vi "Write Power FIFO Direct Dispatch.vi"(4 "T_Out":u64, 6 "T0":u64, 8 "error in (no error)":errorcluster, 9 "Timeout (ms)":i32=100, 10 "Data In":T1[](array[typedef])=[{"measurement"=[], "dT"=0.0, "Timestamp"=0}, {"measurement"=[], "dT"=0.0, "Timestamp"=0}], 11 "CIFTag in":refnum<class "CIFChannels.lvclass">) -> (0 "error out":errorcluster, 1 "timed out?":bool, 2 "Data Out":T1[](array[typedef]), 3 "CIFTag out":refnum<class "CIF_NIChn_Fifo_Power.lvclass">)   [LabVIEW 2021, in "CIF_NIChn_Fifo_Power.lvclass"]
uses:
  CIF_NIChn_Fifo_Power.lvclass
  D:/dev/CIF-LVCore/src/Channels/CIFChannels/CIFChannels.lvclass
  D:/dev/CIF-LVCore/src/Channels/CIF_NIChn/NIChn/CIF_NIChn.lvclass
  CIFChannels/CIFChannels.lvclass
  ChannelCommon/typedef/Datatype Waveform.ctl
  CIFChannels/CIFChannels.lvclass/CIFChannels.ctl
  CIF_NIChn_Fifo_Power.lvclass/CIF_NIChn_Fifo_Power.ctl
  ChannelCommon/CIFFIFO/CIFfifo.lvclass/CIFfifo.ctl
  NIChn/CIF_NIChn.lvclass/CIF_NIChn.ctl
  ChannelCommon/CIFFIFO/Accessors/Read Length.vi
  <vilib>/CIFChannels/SubVIs/Get dll Path.vi
  ChannelCommon/CIFFIFO/Utilities/Update Header.vi
  ChannelCommon/Utilities/Flatten Header.vi
  ChannelCommon/Flatten/Waveform Flatten.vi
  ChannelCommon/CIFFIFO/Accessors/Write T0.vi
  ChannelCommon/CIFFIFO/Accessors/Write T_Out.vi
  ChannelCommon/CIFFIFO/Accessors/Write Payload Length.vi
  ChannelCommon/CIFFIFO/Accessors/Read Header.vi
  ChannelCommon/CIFFIFO/Accessors/Write Header.vi
  CIFChannels/Accessors/Read ClockID.vi
  ChannelCommon/Flatten/Waveform Flatten.vi/e2488641-f297-4923-bbd0-3c2628a14485.vi
  ChannelCommon/Flatten/Waveform Flatten.vi/b4043d5f-ec85-461b-bf30-5d9c9f378a85.vi
  ChannelCommon/Flatten/Waveform Flatten.vi/7a03eb27-3fd6-4af7-b359-0d2263a4e3bc.vi
  CIFCore/Common/Utilities/Append Error Location.vi
  ChannelCommon/Flatten/Waveform Flatten.vi/e2488641-f297-4923-bbd0-3c2628a14485.vi/c28b0ead-42ad-4072-80a2-aca7f2bd7ce3.vi
  ChannelCommon/Flatten/Waveform Flatten.vi/b4043d5f-ec85-461b-bf30-5d9c9f378a85.vi/c28b0ead-42ad-4072-80a2-aca7f2bd7ce3.vi
  ChannelCommon/Flatten/Waveform Flatten.vi/7a03eb27-3fd6-4af7-b359-0d2263a4e3bc.vi/c28b0ead-42ad-4072-80a2-aca7f2bd7ce3.vi
  ChannelCommon/Utilities/Update Time.vi
  NIChn/CIF_NIChn.lvclass
  <vilib>/CIFChannels/CIFChannelCore.lvlib
  ChannelCommon/CIFFIFO/CIFfifo.lvclass
  ChannelCommon/ChannelCommon.lvlib
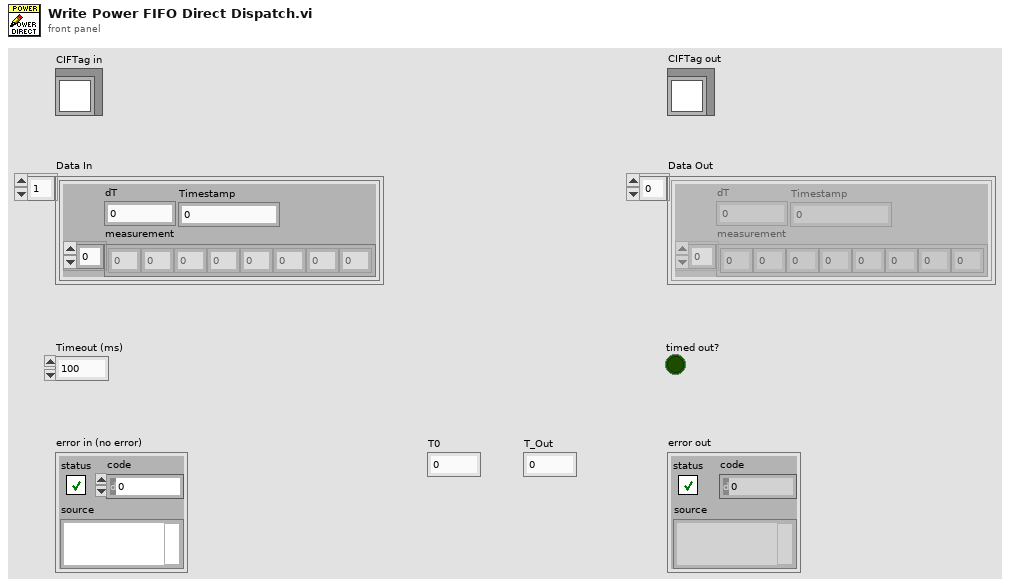
[diagram p1: front panel]
types:
  T1 = typedef "ChannelCommon.lvlib/Datatype Waveform.ctl" = cluster{"measurement":dbl[], "dT":dbl, "Timestamp":u64}
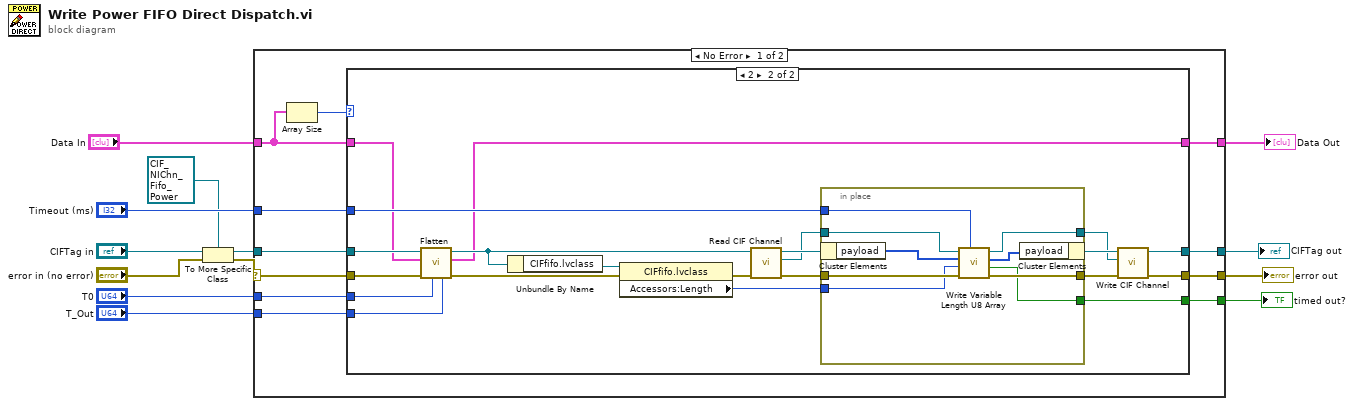
[diagram p0: block diagram]
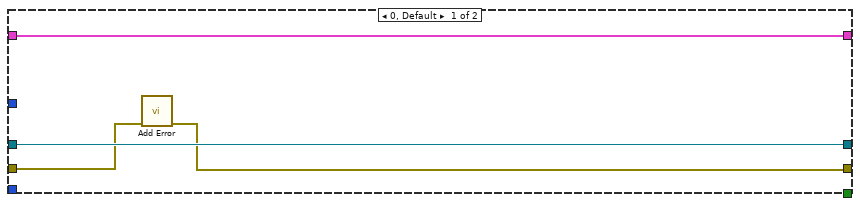
[diagram p2: hidden frame]
diagram:
  n1 = To More Specific Class(target class=refnum<class "CIF_NIChn_Fifo_Power.lvclass"> refnum ("CIFTag in"), reference="CIFTag in", error in="error in (no error)") -> (specific class reference=w5:refnum<class "CIF_NIChn_Fifo_Power.lvclass">, error out=w3:errorcluster)
  n2 = case shown="No Error" w3 {
    selector: w3 -> [w19 w61]
    tunnel: [w21 w61] -> w13
    tunnel: [w23 w60] -> w12
    tunnel: w5 -> [w20 w60]
    tunnel: [w24 _] -> w11
    tunnel: "Timeout (ms)" -> [w22 _]
    tunnel: "T_Out" -> [w17 _]
    tunnel: "T0" -> [w18 _]
    tunnel: "Data In" -> [w14 w59]
    tunnel: [w16 w59] -> w1
    frame No Error {
      n3 = Array Size(array=w14) -> (size(s)=w15:i32)
      n4 = case shown="2" w15 {
        tunnel: [_ w49] -> w24
        tunnel: [w27 w45] -> w23
        tunnel: w22 -> [_ w41]
        tunnel: [w25 w40] -> w21
        tunnel: w20 -> [w27 w37]
        tunnel: w19 -> [w26 w34]
        tunnel: w18 -> [_ w33]
        tunnel: w17 -> [_ w32]
        tunnel: w14 -> [w28 w30]
        tunnel: [w28 w29] -> w16
        frame 0, Default {
          n5 = call "Add Error.vi"("error in (no error)"=w26) -> ("error out"=w25:errorcluster)  [unwired: 10 in]
        }
        frame 2 {
          n6 = call "Flatten.vi"("T_Out"=w32, "T0"=w33, "error in (no error)"=w34, "Data"=w30, "CIFTag in"=w37) -> ("error out"=w35:errorcluster, "Data out"=w29:T1[], "CIFTag out"=w36:refnum<class "CIF_NIChn_Fifo_Power.lvclass">)  [unwired: 4 in]
          n7 = Unbundle By Name(w36) -> ("CIFfifo.lvclass"=w39:refnum<class "CIFfifo.lvclass">)
          n8 = property class="CIFfifo.lvclass"(reference=w39, error in=w35) -> (error out=w38:errorcluster, "Accessors:Length"=w31:u64)  [unwired: 1 out]
          n9 = call "Read CIF Channel.vi"("error in (no error)"=w38, "CIFTag in"=w36) -> ("error out"=w47:errorcluster, "CIF Channel"=w43:refnum<k21>, "CIFTag out"=w48:refnum<class "CIF_NIChn_Fifo_Power.lvclass">)  [unwired: 7 in]
          n10 = in-place {
            in-place-border: w47 -> [w58]
            in-place-border: [w57] -> w44
            in-place-border: [w56] -> w49
            in-place-border: w43 -> [w55]
            in-place-border: [w54] -> w42
            in-place-border: w41 -> [w53]
            in-place-border: w31 -> [w51]
            n11 = in-place-cluster #1(w48) -> ("payload"=w52:u8[])
            n12 = call <vilib>:"Write Variable Length U8 Array.vi"("Timeout (ms)"=w53, "error in"=w58, "numElements"=w51, "U8 Array in"=w52, "CIF Channel in"=w55) -> ("error out"=w57:errorcluster, "Timed out?"=w56:bool, "U8 Array out"=w50:u8[], "CIF Channel out"=w54:refnum<k21>)  [unwired: 3 in]
            n13 = in-place-cluster #1("payload"=w50) -> (w46:refnum<class "CIF_NIChn_Fifo_Power.lvclass">)
          }
          n14 = call "Write CIF Channel.vi"("error in (no error)"=w44, "CIF Channel"=w42, "CIFTag in"=w46) -> ("error out"=w40:errorcluster, "CIFTag out"=w45:refnum<class "CIF_NIChn_Fifo_Power.lvclass">)  [unwired: 7 in]
        }
      }
    }
    frame Error {
    }
  }
  "error out" <- w13
  "CIFTag out" <- w12
  "timed out?" <- w11
  "Data Out" <- w1
